vi "shiftyRegister.vi"() -> ()   [LabVIEW 2016]
panel:
  out "I2":dbl
  out "I":dbl
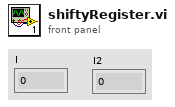
[diagram p1: front panel]
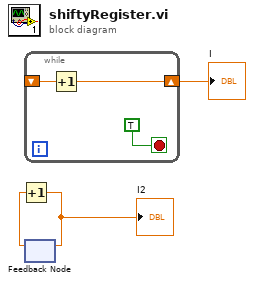
[diagram p0: block diagram]
diagram:
  n1 = while {
    shift-right: [w4] -> w3
    shift-left: _ -> [w5]
    stop <- TRUE stop-if-true
    n2 = Increment(x=w5) -> (x+1=w4:dbl)
  }
  "I" <- w3
  n3 = feedback #1() -> (w1:dbl)  [unwired: 1 in]
  n4 = Increment(x=w1) -> (x+1=w2:dbl)
  "I2" <- w2
  n5 = feedback-in #1(w2) -> ()
